vi "Msg.vi"(7 "Actor in":refnum<class "Actor.lvclass">, 11 "Actor Destroy Msg Strategy in":refnum<class "Actor Destroy Msg Strategy.lvclass">) -> (5 "Actor out":refnum<class "Actor.lvclass">)   [LabVIEW 2021, in "Actor Destroy.lvlib" / "Actor Destroy Msg Strategy.lvclass"]
uses:
  Actor Destroy Msg Strategy.lvclass
  jettl/Actor/Actor.lvclass
  Actor Destroy/Actor Destroy.lvclass
  8b074ebc-55b2-44bc-a317-0de79f881938.vi
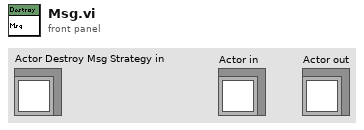
[diagram p1: front panel]
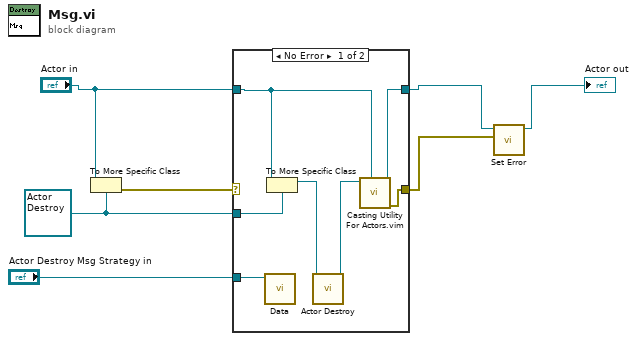
[diagram p0: block diagram]
diagram:
  w4 = refnum<class "Actor Destroy.lvclass"> refnum ("Destroy.lvlib:Destroy.lvclass")
  n1 = To More Specific Class(target class=w4, reference="Actor in") -> (error out=w7:errorcluster)  [unwired: 1 in, 1 out]
  n2 = case shown="No Error" w7 {
    selector: w7 -> [_ w15]
    tunnel: [w13 w16] -> w3
    tunnel: "Actor in" -> [w12 w16]
    tunnel: w4 -> [w14 _]
    tunnel: "Actor Destroy Msg Strategy in" -> [w11 _]
    tunnel: [w8 w15] -> w1
    frame No Error {
      n3 = call "Data.vi"("Actor Destroy Msg Strategy in"=w11) -> ()  [unwired: 11 in]
      n4 = To More Specific Class(target class=w14, reference=w12) -> (specific class reference=w10:refnum<class "Actor Destroy.lvclass">)  [unwired: 1 in, 1 out]
      n5 = call-dynamic "Actor Destroy.vi"("Actor Destroy in"=w10) -> ("Actor Destroy out"=w9:refnum<class "Actor Destroy.lvclass">)  [unwired: 10 in]
      n6 = call "Casting Utility For Actors.vim"("type"=w12, "Actor in"=w9) -> ("error out"=w8:errorcluster, "Actor out"=w13:refnum<class "Actor.lvclass">)  [unwired: 8 in]
    }
    frame Error {
    }
  }
  n7 = call-dynamic "Set Error.vi"("Error"=w1, "Actor in"=w3) -> ("Actor out"=→"Actor out":refnum<class "Actor.lvclass">)  [unwired: 9 in]
